vi "AO 1 Samples FPGA.vi"() -> ()   [LabVIEW 2019]
uses:
  <vilib>/rvi/Emulation/niFpgaGetClockAttributes.vi
  <vilib>/rvi/Emulation/niFpgaSctlEmulationGetInTimedLoop.vi
  <vilib>/rvi/Emulation/niFpgaEmulationReportErrorSimple.vi
  <vilib>/rvi/Emulation/niFpgaEmulationIsFPGAContextNoSignature.vi
  <vilib>/rvi/errors/niFpgaSetErrorForExecOnDevCompSimple.vi
  <vilib>/rvi/eio/common/nirviEmuReportErrorAndStop.vi
  <vilib>/rvi/DataTransferAndStorage/Container/Common/niFpgaContainerGetUniqueNameForEmu.vi
  <vilib>/rvi/FIFO/Fifo_Resource/nirvififoEmulationSetSize.vi
  <vilib>/rvi/FIFO/Fifo_Resource/nirviFifoEmulationQueueMgr.vi
  <instcachedir>/0/nirviFifoEmulationQueueMgr_E5CAEC123FF24DC58D834DCA3CDAA9B5.lvgen/nirviFifoEmulationQueueMgr_E5CAEC123FF24DC58D834DCA3CDAA9B5_004.vi
  <vilib>/rvi/FIFO/Fifo_Resource/nirvififoEmulationDetermineInputValidOut.vi
  <vilib>/rvi/FIFO/Fifo_Resource/nirvififoEmulationCreateLock.vi
  <vilib>/rvi/Emulation/niFpgaProcessEmulError.vi
  <vilib>/rvi/FIFO/Fifo_Resource/nirvififoEmulationObtainLock.vi
  <vilib>/rvi/FIFO/Fifo_Resource/nirvififoEmulationReleaseLock.vi
  <vilib>/rvi/occurrence/nirviWaitOnOccurrenceBase.vi
  <vilib>/rvi/errors/nirviReportUnexpectedCaseInternalError.vi
  <vilib>/rvi/errors/nirviReportUnexpectedCaseInternalError (U32).vi
  <vilib>/rvi/Emulation/niFpgaCriticalErrorInLSC.vi
  <vilib>/Utility/error.llb/Clear Errors.vi
  <vilib>/rvi/eio/common/nirviEmuTemplateMethod_errors.vi
  <vilib>/rvi/DataTransferAndStorage/Container/Common/niFpgaContainerSetEmuInfo.vi
  <vilib>/rvi/DataTransferAndStorage/Container/XNode/niFpgaContainer.xnode
  <vilib>/rvi/FIFO/Fifo_Resource/nirvififoEmulationWrite.vi
  <vilib>/rvi/FIFO/Fifo_Resource/nirvififoEmulationRead.vi
  <vilib>/eio/EIONode/EIONode.xnode
  <vilib>/rvi/LocalResourceManager/LocalResourceManager.xnode
panel:
  in  "开始":bool
  in  "B1.Enable":bool
  in  "B0.Enable":bool
  in  "A1.Enable":bool
  in  "A0.Enable":bool
  in  "B1.Value":fxp<+/-,20,5>
  in  "B0.Value":fxp<+/-,20,5>
  in  "A1.Value":fxp<+/-,20,5>
  in  "A0.Value":fxp<+/-,20,5>
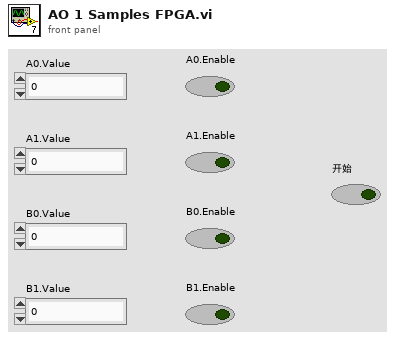
[diagram p1: front panel]
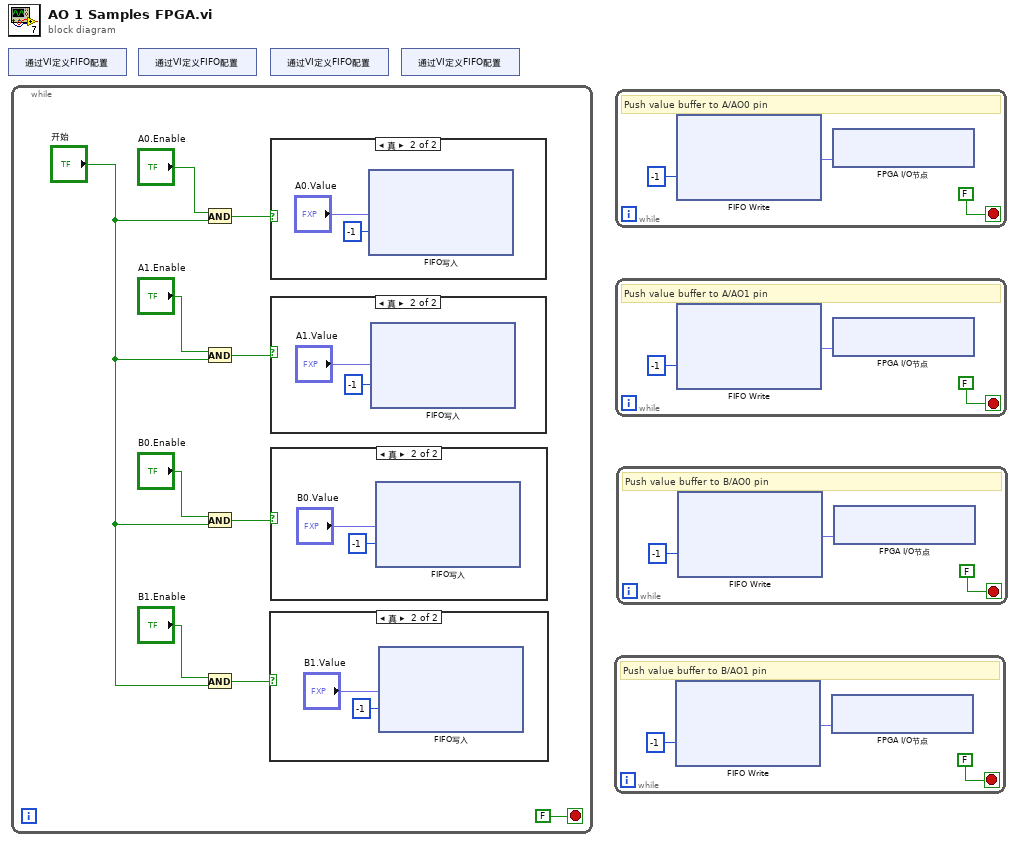
[diagram p0: block diagram]
diagram:
  n1 = xnode "通过VI定义FIFO配置"() -> ()  [unwired: 1 out]
  n2 = while {
    stop <- FALSE stop-if-true
    n3 = And(x="A0.Enable", y="开始") -> (x .and. y?=w10:bool)
    n4 = And(x="A1.Enable", y="开始") -> (x .and. y?=w6:bool)
    n5 = And(x="B0.Enable", y="开始") -> (x .and. y?=w7:bool)
    n6 = And(x="B1.Enable", y="开始") -> (x .and. y?=w8:bool)
    n7 = case shown="真" w8 {
      frame False {
      }
      frame True {
        n8 = xnode "FIFO写入"("元素"="B1.Value", "超时"=-1) -> ()  [unwired: 1 in, 2 out]
      }
    }
    n9 = case shown="真" w10 {
      frame False {
      }
      frame True {
        n10 = xnode "FIFO写入"("元素"="A0.Value", "超时"=-1) -> ()  [unwired: 1 in, 2 out]
      }
    }
    n11 = case shown="真" w6 {
      frame False {
      }
      frame True {
        n12 = xnode "FIFO写入"("元素"="A1.Value", "超时"=-1) -> ()  [unwired: 1 in, 2 out]
      }
    }
    n13 = case shown="真" w7 {
      frame False {
      }
      frame True {
        n14 = xnode "FIFO写入"("元素"="B0.Value", "超时"=-1) -> ()  [unwired: 1 in, 2 out]
      }
    }
  }
  n15 = xnode "通过VI定义FIFO配置"() -> ()  [unwired: 1 out]
  n16 = xnode "通过VI定义FIFO配置"() -> ()  [unwired: 1 out]
  n17 = xnode "通过VI定义FIFO配置"() -> ()  [unwired: 1 out]
  n18 = while {
    stop <- FALSE stop-if-true
    # "Push value buffer to B/AO1 pin"
    n19 = xnode ("FIFO Write")("超时"=-1 ("Timeout")) -> ("元素"=w20:fxp<+/-,20,5>)  [unwired: 1 in, 2 out]
    n20 = xnode "FPGA I/O节点"("ConnectorB/AO1"=w20) -> ()  [unwired: 1 in, 1 out]
  }
  n21 = while {
    stop <- FALSE stop-if-true
    # "Push value buffer to A/AO0 pin"
    n22 = xnode ("FIFO Write")("超时"=-1 ("Timeout")) -> ("元素"=w23:fxp<+/-,20,5>)  [unwired: 1 in, 2 out]
    n23 = xnode "FPGA I/O节点"("ConnectorA/AO0"=w23) -> ()  [unwired: 1 in, 1 out]
  }
  n24 = while {
    stop <- FALSE stop-if-true
    # "Push value buffer to A/AO1 pin"
    n25 = xnode ("FIFO Write")("超时"=-1 ("Timeout")) -> ("元素"=w26:fxp<+/-,20,5>)  [unwired: 1 in, 2 out]
    n26 = xnode "FPGA I/O节点"("ConnectorA/AO1"=w26) -> ()  [unwired: 1 in, 1 out]
  }
  n27 = while {
    stop <- FALSE stop-if-true
    # "Push value buffer to B/AO0 pin"
    n28 = xnode ("FIFO Write")("超时"=-1 ("Timeout")) -> ("元素"=w29:fxp<+/-,20,5>)  [unwired: 1 in, 2 out]
    n29 = xnode "FPGA I/O节点"("ConnectorB/AO0"=w29) -> ()  [unwired: 1 in, 1 out]
  }
